vi "Agilent VNA Set Power Sweep.vi"(8 "error in (no error)":errorcluster, 10 "Start/Stop Power, dBm":cluster{"Pstart":dbl, "Pstop":dbl}, 11 "VISA Resource Name":refnum<visa-resource-name>) -> (0 "error out":errorcluster, 3 "dup VISA Resource Name":refnum<visa-resource-name>)   [LabVIEW 2011]
doc: "This vi sets the power range. Only works on the HP 8753D."
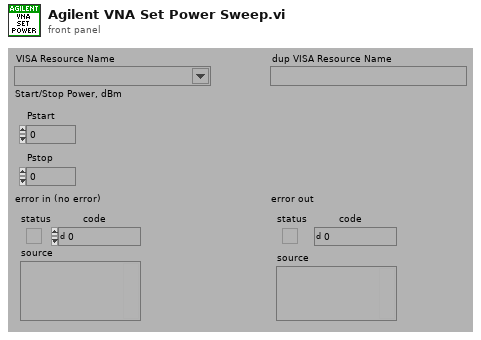
[diagram p1: front panel]
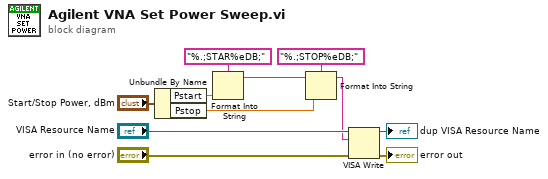
[diagram p0: block diagram]
diagram:
  n1 = Unbundle By Name("Start/Stop Power, dBm") -> ("Pstart"=w3:dbl, "Pstop"=w2:dbl)
  n2 = Format Into String(format string="%.;STAR%eDB;", w3) -> (resulting string=w4:string)  [unwired: 2 in, 1 out]
  n3 = Format Into String(format string="%.;STOP%eDB;", initial string=w4, w2) -> (resulting string=w1:string)  [unwired: 1 in, 1 out]
  n4 = VISA Write(VISA resource name="VISA Resource Name", write buffer=w1, error in (no error)="error in (no error)") -> (VISA resource name out=→"dup VISA Resource Name":refnum<visa-resource-name>, error out=→"error out":errorcluster)  [unwired: 1 out]
